vi "A_4.vi"() -> ()   [LabVIEW 2020]
panel:
  out "Sec counted":string
  in  "stop":bool
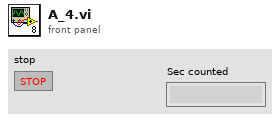
[diagram p1: front panel]
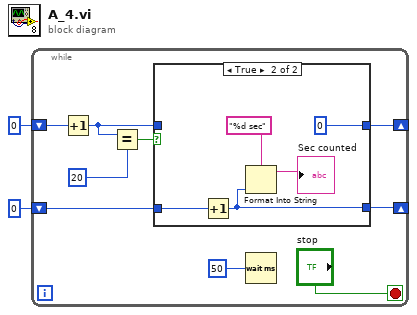
[diagram p0: block diagram]
diagram:
  n1 = while {
    shift-right: [w7] -> _
    shift-left: u32 0 -> [w10]
    shift-right: [w4] -> _
    shift-left: 0 -> [w5]
    stop <- "stop" stop-if-true
    n2 = Increment(x=w10) -> (x+1=w6:u32)
    n3 = Equal?(x=w6, y=u32 20) -> (x = y?=w8:bool)
    n4 = case shown="True" w8 {
      tunnel: [w13 u32 0] -> w7
      tunnel: w6 -> [w13 _]
      tunnel: w5 -> [w12 w18]
      tunnel: [w12 w16] -> w4
      frame False {
      }
      frame True {
        n5 = Increment(x=w18) -> (x+1=w16:i32)
        n6 = Format Into String(format string="%d sec", w16) -> (resulting string=→"Sec counted":string)  [unwired: 2 in, 1 out]
      }
    }
    n7 = Wait (ms)(milliseconds to wait=u32 50) -> ()  [unwired: 1 out]
  }
